vi "连接数据库.vi"(8 "error in (no error)":errorcluster, 10 "数据库连接信息":T1) -> (0 "error out":errorcluster, 3 "obj-数据库操作 o":refnum<class "数据库操作.lvclass">)   [LabVIEW 2013, in "数据库操作.lvclass"]
uses:
  <vilib>/addons/database/Connection.llb/DB Tools Open Connec (String).vi
  <vilib>/addons/database/NI_Database_API.lvlib
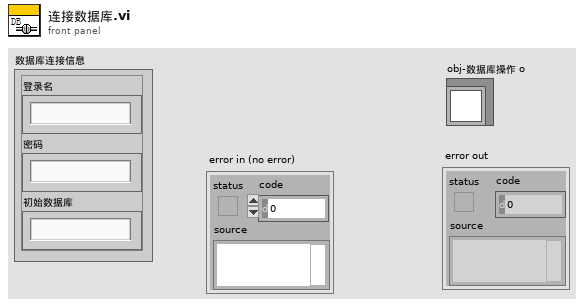
[diagram p1: front panel]
types:
  T1 = cluster{"登录名":string, "密码":string, "初始数据库":string}
  T2 = typedef "NI_Database_API.lvlib/Conn ObjectReference.ctl" = refnum<k1>
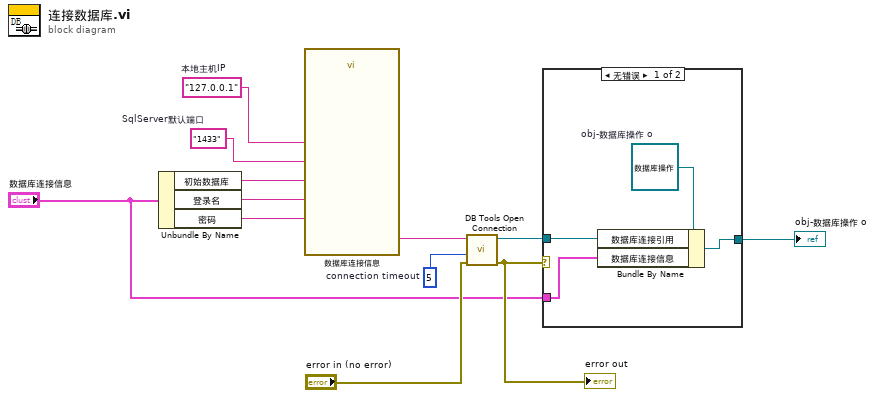
[diagram p0: block diagram]
diagram:
  w2 = "1433"  # SqlServer默认端口
  w3 = "127.0.0.1"  # 本地主机IP
  w11 = 5  # connection timeout
  n1 = Unbundle By Name("数据库连接信息") -> ("初始数据库"=w6:string, "登录名"=w5:string, "密码"=w4:string)
  n2 = call "数据库连接信息"("用户名"=w5, "数据库IP"=w3, "数据库Port"=w2, "初始数据库"=w6, "密码"=w4) -> ("Result"=w12:string)  [unwired: 9 in, 1 out]
  n3 = call-poly <vilib>:"DB Tools Open Connection.vi"("error in (no error)"="error in (no error)", "connection timeout (15)"=w11, "connection information"=w12) -> ("error out"=w10:errorcluster, "connection reference"=w9:T2)  [unwired: 5 in]
  "error out" <- w10
  n4 = case shown="无错误" w10 {
    tunnel: w9 -> [w16 _]
    tunnel: [w15 _] -> w8
    tunnel: "数据库连接信息" -> [w14 _]
    frame No Error {
      w13 = refnum<class "数据库操作.lvclass"> refnum  # obj-数据库操作 o
      n5 = Bundle By Name(cluster=w13, "数据库连接引用"=w16, "数据库连接信息"=w14) -> (w15:refnum<class "数据库操作.lvclass">)
    }
    frame Error {
    }
  }
  "obj-数据库操作 o" <- w8
